vi "Simple Dialog.vi"(9 "Default Value":string, 10 "Prompt":string="Please enter the filename you would like to use.\\n\\nhere:", 11 "Window Title":string="Simple asdfasdfads") -> (2 "OK?":bool=TRUE, 3 "Text Out":string="asdfsdf")   [LabVIEW 2011]
doc: "Simple Dialog box\n\n\nVersion 1.0 - 02/13/2013\n\nPhaeron, Inc.\nwww.phaeron.com\ninfo@phaeron.com"
panel:
  out "Prompt":string
  in  "Value":string
  in  "System Cancel Button":bool
  in  "System OK Button":bool
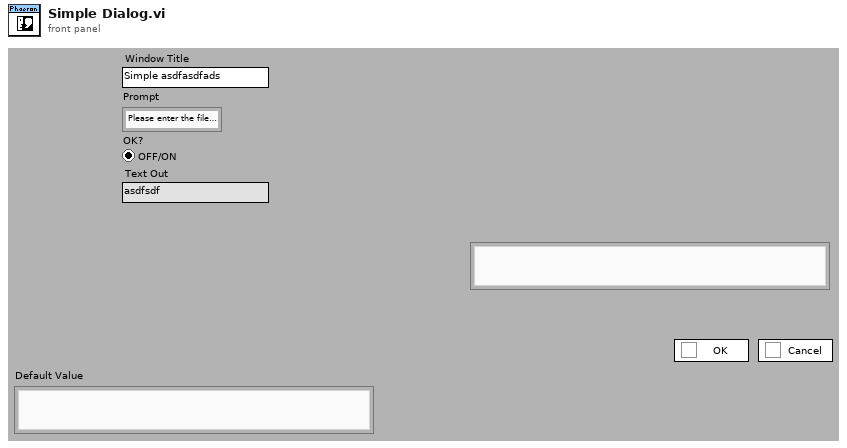
[diagram p1: front panel]
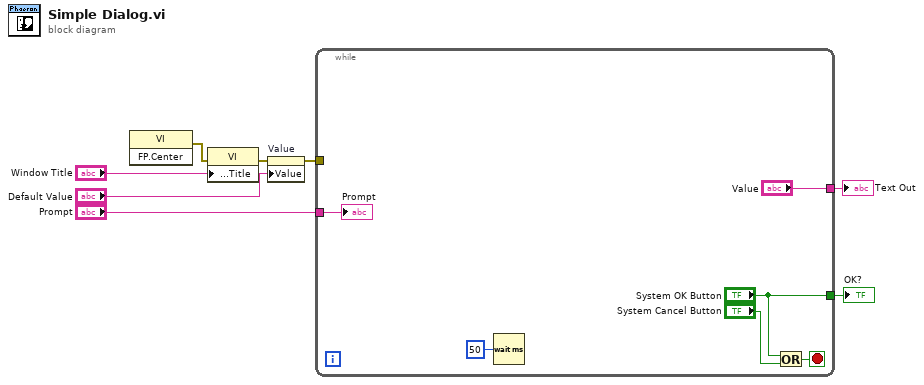
[diagram p0: block diagram]
diagram:
  n1 = invoke class="VI" method="FP.Center"() -> (error out=w2:errorcluster)  [unwired: 3 in, 2 out]
  n2 = property class="VI"(error in=w2, "Front Panel.Title"="Window Title") -> (error out=w4:errorcluster)  [unwired: 1 in, 1 out]
  n3 = property on="Value" class="Str"(error in=w4, "Value"="Default Value") -> (error out=w3:errorcluster)  [unwired: 1 in, 1 out]
  n4 = while {
    tunnel: ["Value"] -> w7
    tunnel: ["System OK Button"] -> w6
    tunnel: w3 -> [_]
    tunnel: "Prompt" -> [w9]
    stop <- w13 stop-if-true
    n5 = Wait (ms)(milliseconds to wait=u32 50) -> ()  [unwired: 1 out]
    n6 = Or(x="System OK Button", y="System Cancel Button") -> (x .or. y?=w13:bool)
    "Prompt" <- w9
  }
  "Text Out" <- w7
  "OK?" <- w6
